vi "Log Error.vi"(8 "error in (no error)":errorcluster, 10 "Error Message Data":T1, 11 "Text Log In":refnum<class "Text Log.lvclass">) -> (0 "error out":errorcluster, 3 "Text Log Out":refnum<class "Text Log.lvclass">)   [LabVIEW 2020, in "Error Log Classes.lvlib" / "Text Log.lvclass"]
uses:
  Text Log.lvclass
  Process Classes/Error Handler/Public/TypeDefs/Error Message Data.ctl
  Process Classes/Error Handler/Error Handler.lvclass
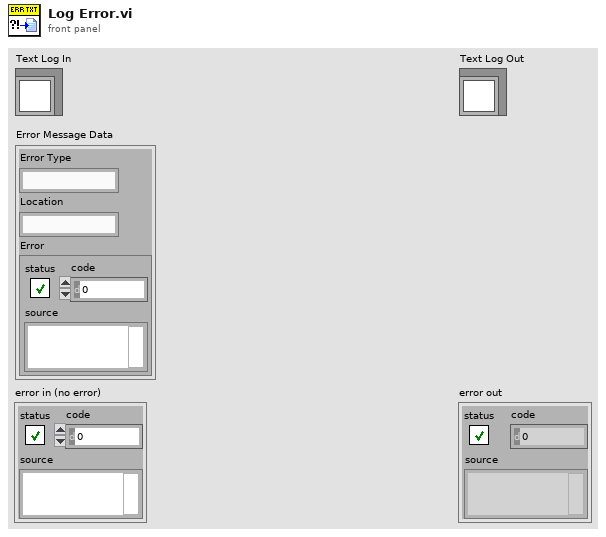
[diagram p1: front panel]
types:
  T1 = typedef "Error Handler.lvclass/Error Message Data.ctl" = cluster{"Error Type":string, "Location":string, "Error":errorcluster}
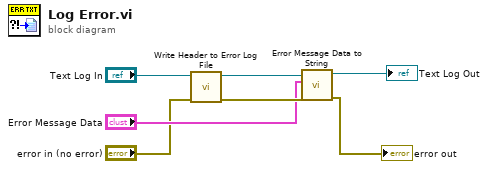
[diagram p0: block diagram]
diagram:
  n1 = call "Write Header to Error Log File.vi"("error in (no error)"="error in (no error)", "Text Log In"="Text Log In") -> ("error out"=w6:errorcluster, "Text Log Out"=w7:refnum<class "Text Log.lvclass">)  [unwired: 8 in]
  n2 = call "Error Message Data to String.vi"("error in (no error)"=w6, "Error Message Data"="Error Message Data", "Text Log In"=w7) -> ("error out"=→"error out":errorcluster, "Text Log Out"=→"Text Log Out":refnum<class "Text Log.lvclass">)  [unwired: 7 in]
